vi "Dequeue Message.vi"(8 "error in (no error)":errorcluster, 9 "timeout in ms (-1)":i32=-1, 11 "Process In":refnum<class "Process.lvclass">) -> (0 "error out":errorcluster, 1 "Message Data":variant, 2 "Message":string, 3 "Process Out":refnum<class "Process.lvclass">)   [LabVIEW 2020, in "Process.lvclass"]
doc: "This VI pulls messages off the Message Queue."
uses:
  Process.lvclass
  Process.lvclass/Process.ctl
  <vilib>/Utility/error.llb/Error Cluster From Error Code.vi
  <vilib>/ErrorRing/Error Ring.xnode
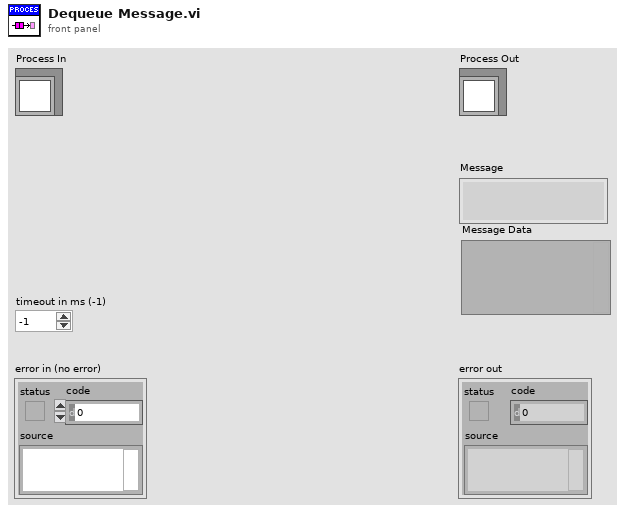
[diagram p1: front panel]
types:
  T1 = typedef "Process.lvclass/Message Cluster.ctl" = cluster{"Message":string, "Message Data":variant, "Request Notifier":refnum<notifier>}
  T2 = cluster{"Action":string, "Call Chain":string, "Process":string, "Message":string, "Message Data":variant, "Time":u32}
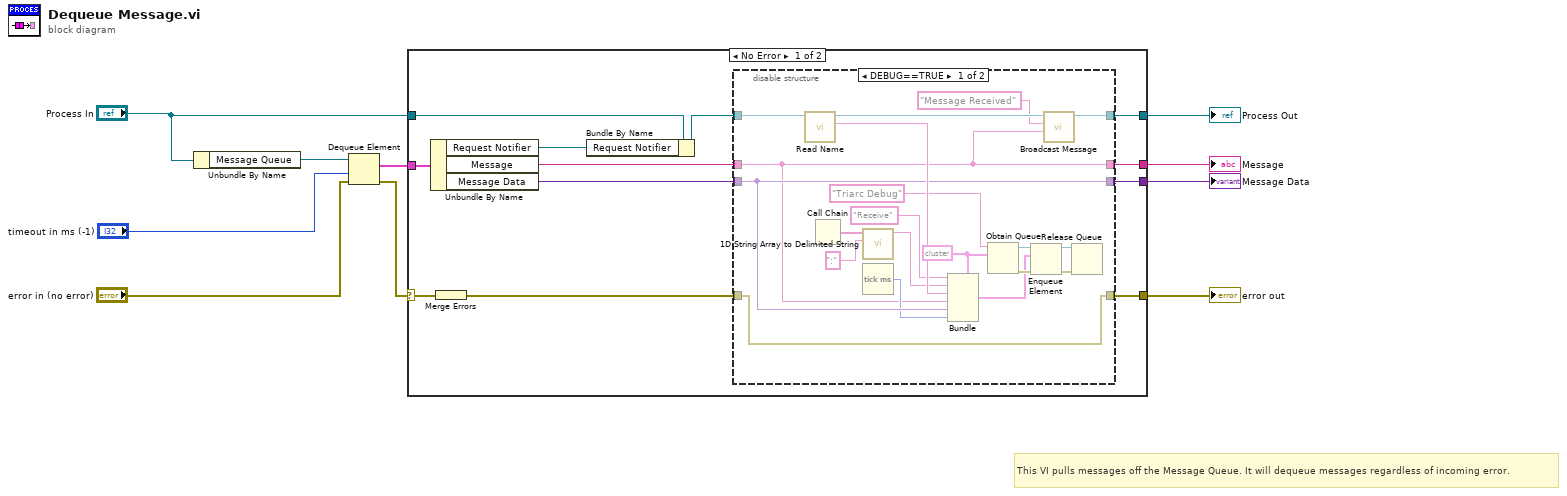
[diagram p0: block diagram]
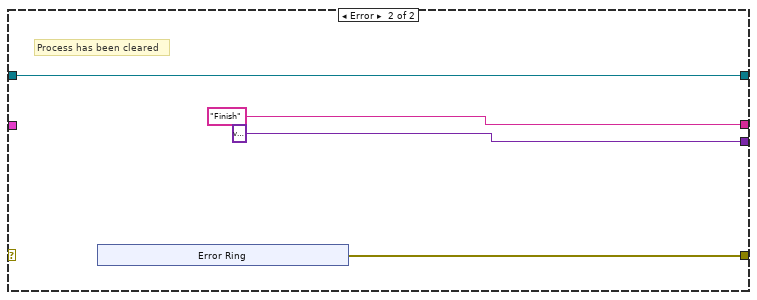
[diagram p3: hidden frame]
diagram:
  # "This VI pulls messages off the Message Queue. It will dequeue messages regardless of incoming error."
  n1 = Unbundle By Name("Process In") -> ("Message Queue"=w10:refnum<queue>)
  n2 = Dequeue Element(queue=w10, timeout in ms (-1)="timeout in ms (-1)", error in (no error)="error in (no error)") -> (element=w4:T1, error out=w5:errorcluster)  [unwired: 2 out]
  n3 = case shown="No Error" w5 {
    selector: w5 -> [w22 _]
    tunnel: [w14 w48] -> w9
    tunnel: [w17 "Finish" ("Message")] -> w8
    tunnel: [w18 variant ("Message Data")] -> w7
    tunnel: w4 -> [w21 _]
    tunnel: [w16 w47] -> w1
    tunnel: "Process In" -> [w15 w47]
    frame No Error {
      n4 = Unbundle By Name(w21) -> ("Request Notifier"=w11:refnum<notifier>, "Message"=w20:string, "Message Data"=w19:variant)
      n5 = Merge Errors(w22) -> (w13:errorcluster)
      n6 = Bundle By Name(cluster=w15, "Request Notifier"=w11) -> (w12:refnum<class "Process.lvclass">)
      n7 = disable-structure shown="DEBUG==TRUE" {
        disable-tunnel: w20 -> [w23 w46]
        disable-tunnel: w19 -> [w29 w45]
        disable-tunnel: [w29 w45] -> w18
        disable-tunnel: [w23 w46] -> w17
        disable-tunnel: [w25 w44] -> w16
        disable-tunnel: w12 -> [w27 w44]
        disable-tunnel: [w30 w43] -> w14
        disable-tunnel: w13 -> [w30 w43]
        frame condition #0 {
          w37 = T2 {"Action"="", "Call Chain"="", "Process"="", "Message"="", "Message Data"=variant, "Time"=0} ("output cluster")
          n8 = call-dynamic "Read Name.vi"("Process In"=w27) -> ("Qualified Name"=w42:string, "Process Out"=w28:refnum<class "Process.lvclass">)  [unwired: 7 in, 2 out]
          n9 = Call Chain() -> (call chain=w41:string[])
          n10 = call <vilib>:"1D String Array to Delimited String.vi"("delimiter"=":", "string array"=w41) -> ("delimited string"=w39:string)  [unwired: 9 in]
          n11 = Tick Count (ms)() -> (millisecond timer value=w26:u32)
          n12 = Bundle(cluster=w37, "Action"="Receive", "Call Chain"=w39, "Process"=w42, "Message"=w23, "Message Data"=w29, "Time"=w26) -> (w34:T2)
          n13 = Obtain Queue(name (unnamed)="Triarc Debug", element data type=w37) -> (queue out=w36:refnum<queue>, error out=w35:errorcluster)  [unwired: 3 in, 1 out]
          n14 = Enqueue Element(queue=w36, element=w34, error in (no error)=w35) -> (queue out=w33:refnum<queue>, error out=w32:errorcluster)  [unwired: 1 in, 1 out]
          n15 = call-dynamic "Broadcast Message.vi"("Message Data"=w23, "Message"="Message Received" ("name (unnamed)"), "Rig Process In"=w28) -> ("Rig Process Out"=w25:refnum<class "Process.lvclass">)  [unwired: 7 in, 1 out]
          n16 = Release Queue(queue=w33, error in (no error)=w32) -> ()  [unwired: 1 in, 3 out]
        }
        frame condition #1 (active) {
        }
      }
    }
    frame Error {
      # "Process has been cleared"
      n17 = xnode "Error Ring"() -> ("error out"=w48:errorcluster)
    }
  }
  "error out" <- w9
  "Process Out" <- w1
  "Message" <- w8
  "Message Data" <- w7
